vi "NewLogFilesComplete Event Callback.vi"(4 "New File Complete":refnum<user-event>, 5 "Event Data":cluster{"sender":refnum<k24>, "e":refnum<k24>}, 6 "Control Ref":refnum<k24>, 7 "Event Common Data":T1) -> ()   [LabVIEW 2020, in "NI_VS Data Logging API.lvlib"]
uses:
  <vilib>/NI VeriStand/Execution/DataLogging/NI_VS Data Logging API.lvlib
  NationalInstruments.VeriStand.ClientAPI
  <vilib>/NI VeriStand/Execution/DataLogging/New Log Files Complete Event Data.ctl
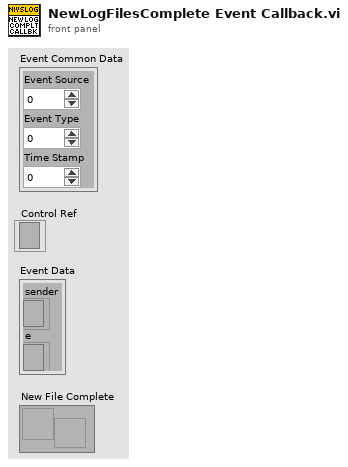
[diagram p1: front panel]
types:
  T1 = cluster{"Event Source":i32, "Event Type":u32, "Time Stamp":u32}
  T2 = typedef "NI_VS Data Logging API.lvlib/New Log Files Complete Event Data.ctl" = cluster{"Log File Paths":path[], "Log File Source":string, "Target":string}
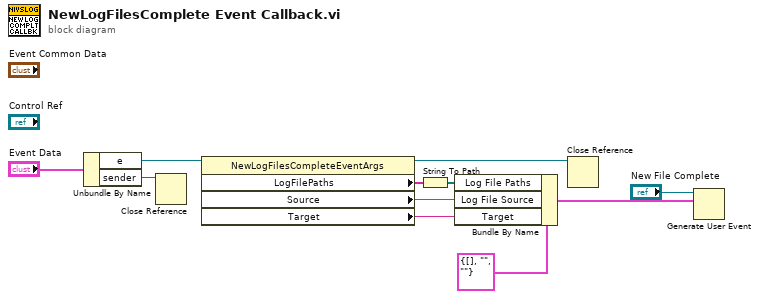
[diagram p0: block diagram]
diagram:
  n1 = Unbundle By Name("Event Data") -> ("e"=w9:refnum<k24>, "sender"=w2:refnum<k24>)
  n2 = Close Reference(reference=w2) -> ()  [unwired: 1 in, 1 out]
  n3 = property class="NewLogFilesCompleteEventArgs"(reference=w9) -> (reference out=w8:refnum<k24>, "LogFilePaths"=w6:string[], "Source"=w4:string, "Target"=w1:string)  [unwired: 1 in, 1 out]
  n4 = String To Path(string=w6) -> (path=w5:path[])
  n5 = Bundle By Name(cluster=T2 {"Log File Paths"=[], "Log File Source"="", "Target"=""} ("New Log File Complete Event Data"), "Log File Paths"=w5, "Log File Source"=w4, "Target"=w1) -> (w3:T2)
  n6 = Close Reference(reference=w8) -> ()  [unwired: 1 in, 1 out]
  n7 = Generate User Event(user event="New File Complete", event data cluster=w3) -> ()  [unwired: 2 in, 2 out]
